vi "z_control_statemachine_FP.vi"(4 "Kiz_down":sgl format="%#_13g", 5 "uz_safe":fxp<+/-,16,5>, 6 "z-axis-params":T1={"TOL"=0.3, "ramp_rate"=0.0, "z_u_max"=5.0, "setpoint"=0.0, "Ki"=0.001, "Z_error_threshold"=0.0, "Z_settled_samples_threshold "=0, "z_UP"=0.0, "zup_N"=0, "TF Order"=2, "Num"=[-0.00254, 0.000408, 0.00295, 0.0, 0.0, 0.0, 0.0, 0.0, 0.0], "Den"=[0.982758, -1.98194, 1.0, 0.0, 0.0, 0.0, 0.0, 0.0, 0.0]} {"Z_error_threshold" format="%#_13g"; "ramp_rate" format="%#_13g"; "TOL" format="%#_13g"}, 7 "zup_rate":sgl, 8 "step_down_frac":fxp<+,8,1>, 9 "init Z up":fxp<+/-,16,5>, 10 "State":u8, 11 "zerr(k)":sgl) -> (3 "z-u(k)":fxp<+/-,16,5>)   [LabVIEW 2017]
uses:
  z-axis-params.ctl
  <vilib>/rvi/Emulation/niFpgaEmulationIsFPGAContextNoSignature.vi
  <vilib>/rvi/DataTransferAndStorage/Container/Common/niFpgaContainerGetUniqueNameForEmu.vi
  <vilib>/rvi/Memory/Memory_Emulation/niFpgaMemoryEmulationCacheClearOnFirstRun.vi
  <vilib>/rvi/Memory/Memory_Emulation/nirvimemoryEmulationManagerCache_MakeExclusive.vi
  <vilib>/rvi/Memory/Memory_Emulation/niFpgaMemoryEmulationValidateCache.vi
  <vilib>/rvi/Memory/Memory_Emulation/nirvimemoryEmulationManagerCache_InsertValue.vi
  <vilib>/Utility/error.llb/Clear Errors.vi
  <vilib>/rvi/Memory/Memory_Emulation/nirvimemoryEmulationManagerCache_ReleaseExclusive.vi
  <vilib>/rvi/Memory/Memory_Emulation/nirvimemoryEmulationManagerCache_GetValue.vi
  <vilib>/rvi/Memory/Memory_Emulation/nirvimemoryEmulationManagerCache_SetValue.vi
  <vilib>/rvi/Emulation/niFpgaProcessEmulError.vi
  <vilib>/rvi/Emulation/niFpgaSctlEmulationGetInTimedLoop.vi
  <vilib>/rvi/DataTransferAndStorage/Container/XNode/niFpgaContainer.xnode
  <vilib>/rvi/DataTransferAndStorage/Register/Emulation/niFpgaRegisterEmulation.vi
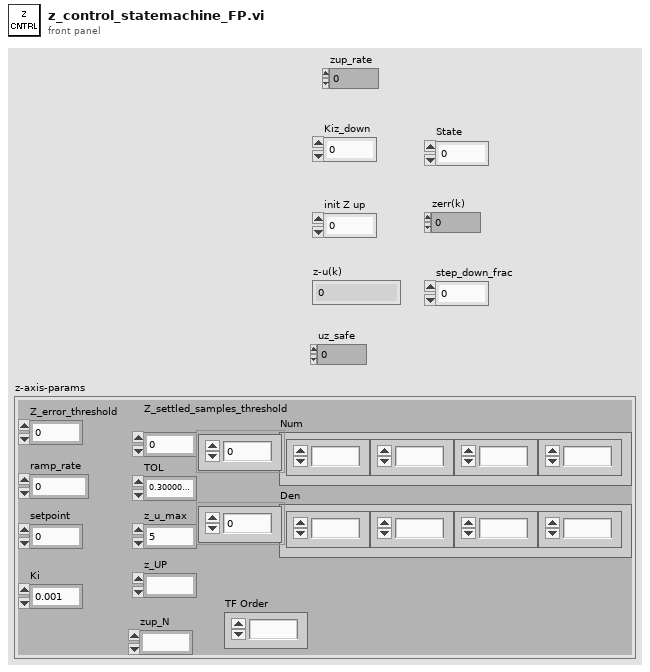
[diagram p1: front panel]
types:
  T1 = typedef "z-axis-params.ctl" = cluster{"TOL":sgl, "ramp_rate":sgl, "z_u_max":sgl, "setpoint":sgl, "Ki":sgl, "Z_error_threshold":sgl, "Z_settled_samples_threshold ":i16, "z_UP":fxp<+/-,16,5>, "zup_N":i16, "TF Order":i32, "Num":sgl[], "Den":sgl[]}
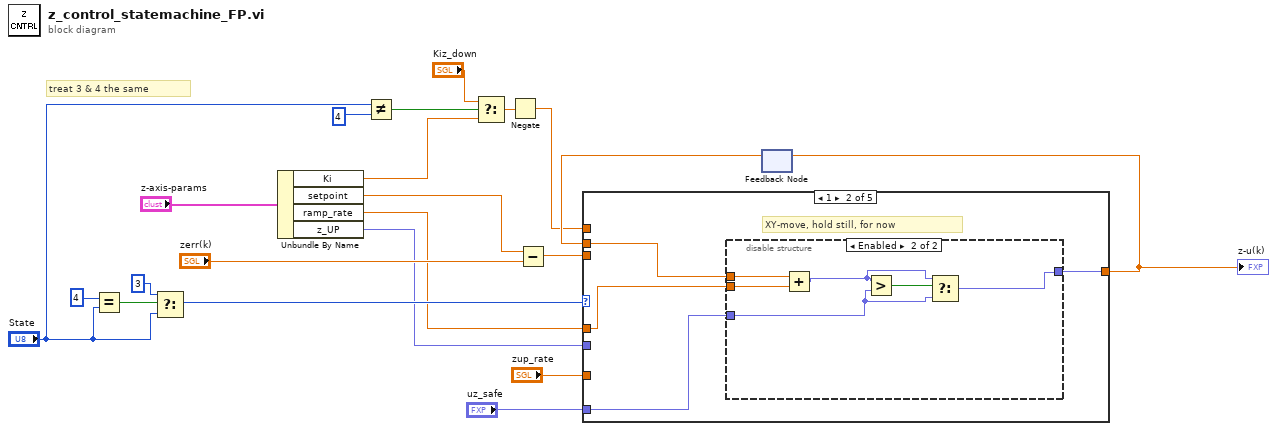
[diagram p0: block diagram]
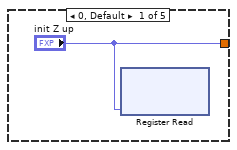
[diagram p2: hidden frame]
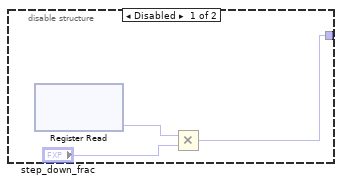
[diagram p3: hidden frame]
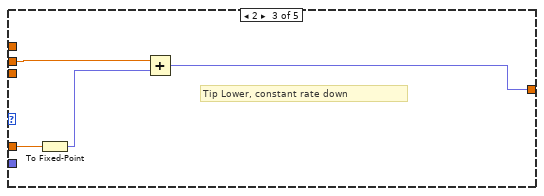
[diagram p4: hidden frame]
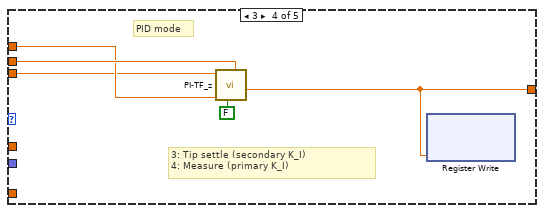
[diagram p5: hidden frame]
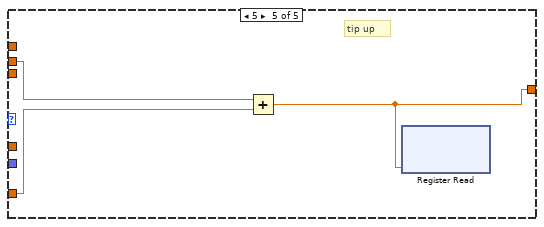
[diagram p6: hidden frame]
diagram:
  # "treat 3 & 4 the same"
  n1 = Equal?(x=i8 4 ("y"), y="State") -> (x = y?=w13:bool)
  n2 = Select(t=i8 3 ("y"), s=w13, f="State") -> (s? t:f=w11:u8)
  n3 = Unbundle By Name("z-axis-params") -> ("Ki"=w6:sgl, "setpoint"=w5:sgl, "ramp_rate"=w4:sgl, "z_UP"=w3:fxp<+/-,16,5>)
  n4 = Not Equal?(x="State", y=i8 4) -> (x != y?=w20:bool)
  n5 = Select(t="Kiz_down", s=w20, f=w6) -> (s? t:f=w19:sgl)
  n6 = Negate(x=w19) -> (-x=w15:sgl)
  n7 = Subtract(x=w5, y="zerr(k)") -> (x-y=w14:sgl)
  n8 = feedback #1() -> (w16:sgl)  [unwired: 1 in]
  n9 = case shown="1" w11 {
    tunnel: ["init Z up" w26 w38 w40 w45] -> w10
    tunnel: w16 -> [_ w23 w36 w43 w47]
    tunnel: w15 -> [_ _ _ w42 _]
    tunnel: w14 -> [_ _ _ w41 _]
    tunnel: w4 -> [_ w24 w39 _ _]
    tunnel: w3 -> [_ _ _ _ _]
    tunnel: "zup_rate" -> [_ _ _ _ w46]
    tunnel: "uz_safe" -> [_ w25 _ _ _]
    frame 0, Default {
      n10 = xnode ("Register Read")("Data"="init Z up") -> ()  [unwired: 1 in, 1 out]
    }
    frame 1 {
      # "XY-move, hold still, for now"
      n11 = disable-structure shown="Enabled" {
        disable-tunnel: [w27 w33] -> w26
        disable-tunnel: w25 -> [_ w32]
        disable-tunnel: w24 -> [_ w31]
        disable-tunnel: w23 -> [_ w30]
        frame Disabled {
          n12 = xnode ("Register Read")() -> ("Data"=w28:fxp<+/-,16,5>)  [unwired: 1 in, 1 out]
          n13 = Multiply(x=w28, y="step_down_frac") -> (x*y=w27:fxp<+/-,24,6>)
        }
        frame Enabled {
          n14 = Add(x=w30, y=w31) -> (x+y=w34:fxp<+/-,16,5>)
          n15 = Greater?(x=w34, y=w32) -> (0:w35:bool)
          n16 = Select(t=w34, s=w35, f=w32) -> (s? t:f=w33:fxp<+/-,16,5>)
        }
      }
    }
    frame 2 {
      # "Tip Lower, constant rate down"
      n17 = To Fixed-Point(number=w39) -> (fixed-point=w37:fxp<+/-,16,5>)  [unwired: 1 in]
      n18 = Add(x=w36, y=w37) -> (x+y=w38:fxp<+/-,16,5>)
    }
    frame 3 {
      # "3: Tip settle (secondary K_I)\n4: Measure (primary K_I)"
      # "PID mode"
      n19 = call "PI-TF_z.vi"("u(k-1)"=w43, "reset"=FALSE, "Ki"=w42, "e(k)"=w41) -> ("u(k)"=w40:sgl)  [unwired: 7 in]
      n20 = xnode ("Register Write")("Data"=w40) -> ()  [unwired: 1 in, 1 out]
    }
    frame 5 {
      # "tip up"
      n21 = Add(x=w47, y=w46) -> (x+y=w45:sgl)
      n22 = xnode ("Register Read")("Data"=w45) -> ()  [unwired: 1 in, 1 out]
    }
  }
  "z-u(k)" <- w10
  n23 = feedback-in #1(w10) -> ()
